vi "黑白棋.vi"() -> ()   [LabVIEW 2021]
panel:
  out "下棋者顏色":bool
  out "回合":dbl
  in  "停止":bool
  in  "開始":bool
  in  "Boolean 57":bool
  in  "Boolean 58":bool
  in  "Boolean 59":bool
  in  "Boolean 60":bool
  in  "Boolean 61":bool
  in  "Boolean 62":bool
  in  "Boolean 63":bool
  in  "Boolean 64":bool
  in  "Boolean 49":bool
  in  "Boolean 50":bool
  in  "Boolean 51":bool
  in  "Boolean 52":bool
  in  "Boolean 53":bool
  in  "Boolean 54":bool
  in  "Boolean 55":bool
  in  "Boolean 56":bool
  in  "Boolean 41":bool
  in  "Boolean 42":bool
  in  "Boolean 43":bool
  in  "Boolean 44":bool
  in  "Boolean 45":bool
  in  "Boolean 46":bool
  in  "Boolean 47":bool
  in  "Boolean 48":bool
  in  "Boolean 33":bool
  in  "Boolean 34":bool
  in  "Boolean 35":bool
  in  "Boolean 36":bool
  in  "Boolean 37":bool
  in  "Boolean 38":bool
  in  "Boolean 39":bool
  in  "Boolean 40":bool
  in  "Boolean 25":bool
  in  "Boolean 26":bool
  in  "Boolean 27":bool
  in  "Boolean 28":bool
  in  "Boolean 29":bool
  in  "Boolean 30":bool
  in  "Boolean 31":bool
  in  "Boolean 32":bool
  in  "Boolean 17":bool
  in  "Boolean 18":bool
  in  "Boolean 19":bool
  in  "Boolean 20":bool
  in  "Boolean 21":bool
  in  "Boolean 22":bool
  in  "Boolean 23":bool
  in  "Boolean 24":bool
  in  "Boolean 9":bool
  in  "Boolean 10":bool
  in  "Boolean 11":bool
  in  "Boolean 12":bool
  in  "Boolean 13":bool
  in  "Boolean 14":bool
  in  "Boolean 15":bool
  in  "Boolean 16":bool
  in  "Boolean 8":bool
  in  "Boolean 7":bool
  in  "Boolean 6":bool
  in  "Boolean 5":bool
  in  "Boolean 4":bool
  in  "Boolean 3":bool
  in  "Boolean 2":bool
  in  "Boolean":bool
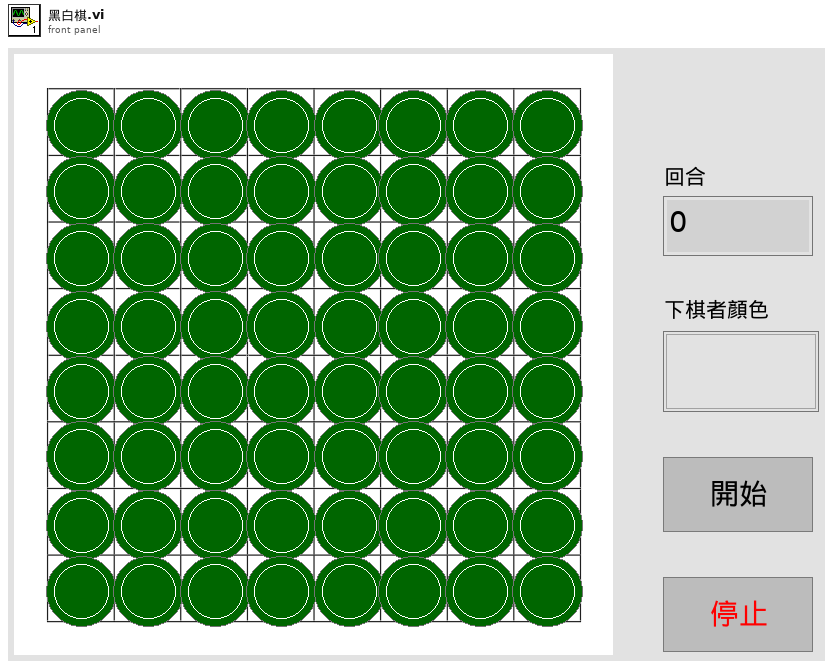
[diagram p1: front panel]
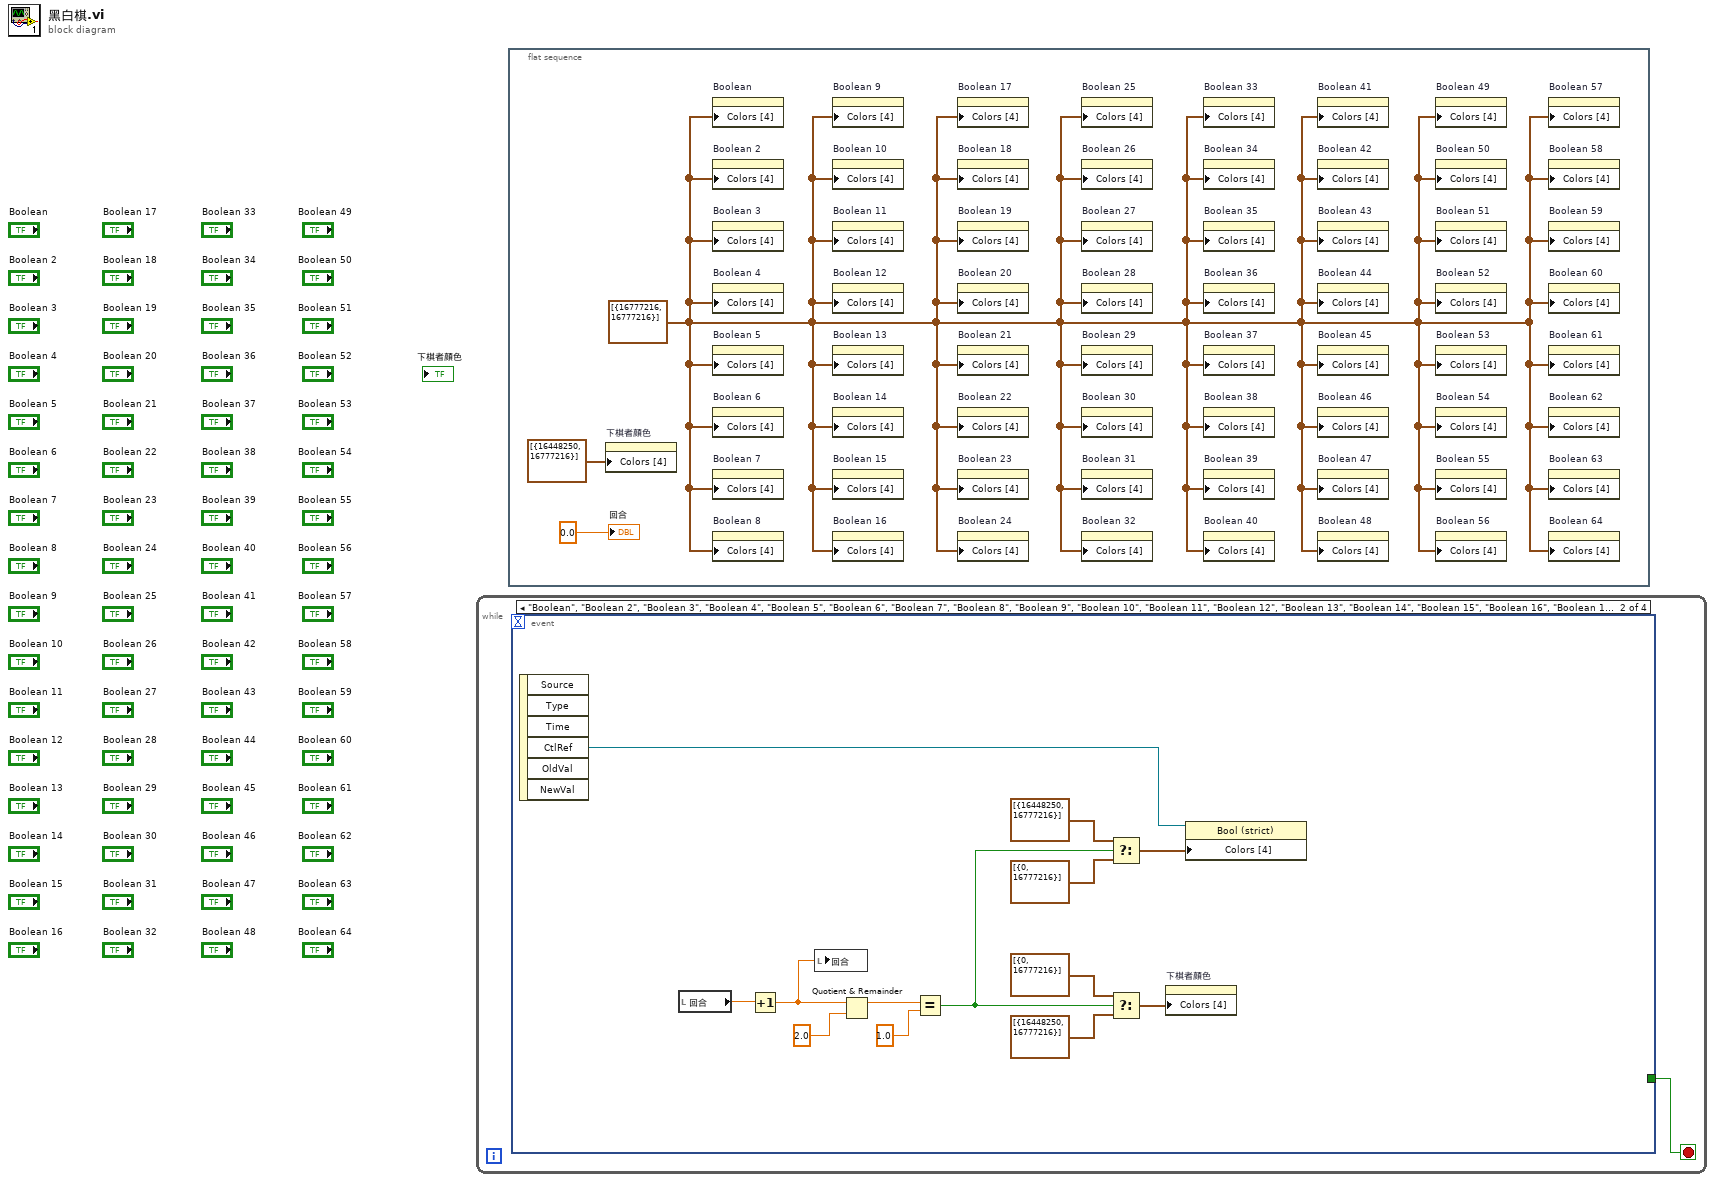
[diagram p0: block diagram]
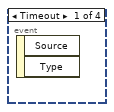
[diagram p2: hidden frame]
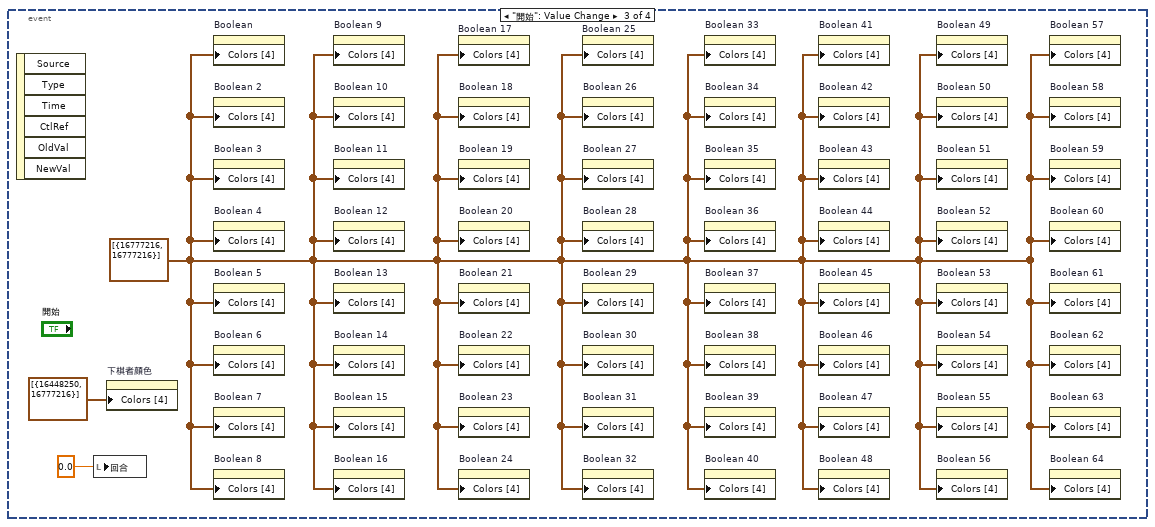
[diagram p3: hidden frame]
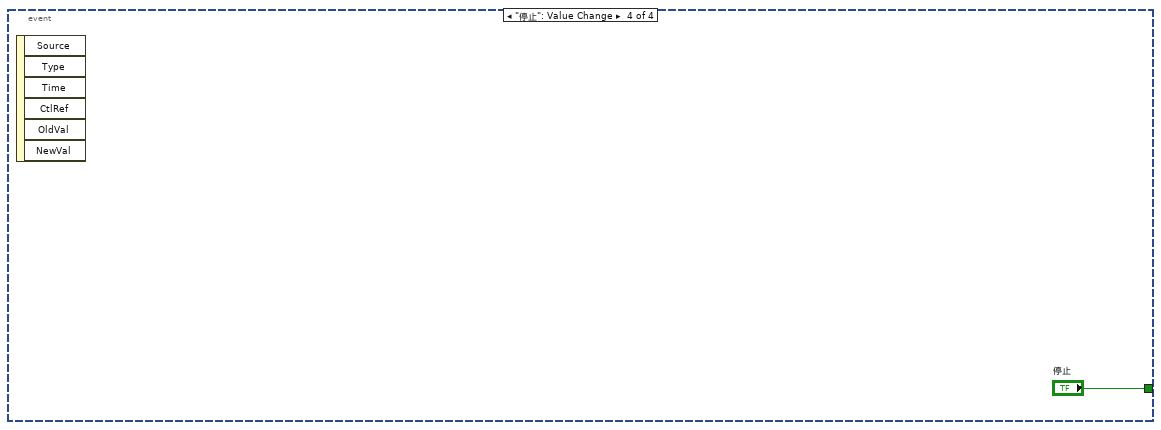
[diagram p4: hidden frame]
diagram:
  n1 = while {
    stop <- w1 stop-if-true
    n2 = event shown="[1] \"Boolean\", \"Boolean 2\", \"Boolean 3\", \"Boolean 4\", \"Boolean 5\", \"Boolean 6\", \"Boolean 7\", \"Boolean 8\", \"Boolean 9\", \"Boolean 10\", \"Boolean 11\", \"Boolean 12\", \"Boolean 13\", \"Boolean 14\", \"Boolean 15\", \"Boolean 16\", \"Boolean 17\", \"Boolean 18\", \"Boolean 19\", \"Boolean 20\", \"Boolean 21\", \"Boolean 22\", \"Boolean 23\", \"Boolean 24\", \"Boolean 25\", \"Boolean 26\", \"Boolean 27\", \"Boolean 28\", \"Boolean 29\", \"Boolean 30\", \"Boolean 31\", \"Boolean 32\", \"Boolean 33\", \"Boolean 34\", \"Boolean 35\", \"Boolean 36\", \"Boolean 37\", \"Boolean 38\", \"Boolean 39\", \"Boolean 40\", \"Boolean 41\", \"Boolean 42\", \"Boolean 43\", \"Boolean 44\", \"Boolean 45\", \"Boolean 46\", \"Boolean 47\", \"Boolean 48\", \"Boolean 49\", \"Boolean 50\", \"Boolean 51\", \"Boolean 52\", \"Boolean 53\", \"Boolean 54\", \"Boolean 55\", \"Boolean 56\", \"Boolean 57\", \"Boolean 58\", \"Boolean 59\", \"Boolean 60\", \"Boolean 61\", \"Boolean 62\", \"Boolean 63\", \"Boolean 64\": Value Change" {
      selector: _ -> [_ _ _ _]
      dyn-events: _ -> [_ _ _ _]
      timeout: _ -> [_ _ _ _]
      tunnel: [_ _ _ "停止"] -> w1
      event Timeout {
        n3 = event-data() -> ()  [unwired: 1 in, 2 out]
      }
      event "Boolean", "Boolean 2", "Boolean 3", "Boolean 4", "Boolean 5", "Boolean 6", "Boolean 7", "Boolean 8", "Boolean 9", "Boolean 10", "Boolean 11", "Boolean 12", "Boolean 13", "Boolean 14", "Boolean 15", "Boolean 16", "Boolean 17", "Boolean 18", "Boolean 19", "Boolean 20", "Boolean 21", "Boolean 22", "Boolean 23", "Boolean 24", "Boolean 25", "Boolean 26", "Boolean 27", "Boolean 28", "Boolean 29", "Boolean 30", "Boolean 31", "Boolean 32", "Boolean 33", "Boolean 34", "Boolean 35", "Boolean 36", "Boolean 37", "Boolean 38", "Boolean 39", "Boolean 40", "Boolean 41", "Boolean 42", "Boolean 43", "Boolean 44", "Boolean 45", "Boolean 46", "Boolean 47", "Boolean 48", "Boolean 49", "Boolean 50", "Boolean 51", "Boolean 52", "Boolean 53", "Boolean 54", "Boolean 55", "Boolean 56", "Boolean 57", "Boolean 58", "Boolean 59", "Boolean 60", "Boolean 61", "Boolean 62", "Boolean 63", "Boolean 64": Value Change {
        n4 = event-data() -> ("CtlRef"=w2:refnum<vi>)  [unwired: 1 in, 5 out]
        n5 = local read "回合"() -> (w14:dbl)
        n6 = Increment(x=w14) -> (x+1=w12:dbl)
        n7 = local write "回合"(w12) -> ()
        n8 = Quotient & Remainder(x=w12, y=2.0) -> (x-y*floor(x/y)=w11:dbl)  [unwired: 1 out]
        n9 = Equal?(x=w11, y=1.0) -> (x = y?=w3:bool)
        n10 = Select(t=cluster{u32, u32}[] [{16448250, 16777216}] ("Colors [4]"), s=w3, f=cluster{u32, u32}[] [{0, 16777216}] ("Colors [4]")) -> (s? t:f=w4:cluster{u32, u32}[])
        n11 = Select(t=cluster{u32, u32}[] [{0, 16777216}] ("Colors [4]"), s=w3, f=cluster{u32, u32}[] [{16448250, 16777216}] ("Colors [4]")) -> (s? t:f=w7:cluster{u32, u32}[])
        n12 = property on="下棋者顏色" class="Bool (strict)"("Colors [4]"=w7) -> ()  [unwired: 2 in, 2 out]
        n13 = property class="Bool (strict)"(reference=w2, "Colors [4]"=w4) -> ()  [unwired: 1 in, 2 out]
      }
      event "開始": Value Change {
        w15 = cluster{u32, u32}[] [{16777216, 16777216}] ("Colors [4]")
        n14 = event-data() -> ()  [unwired: 1 in, 6 out]
        n15 = local write "回合"(0.0 ("回合")) -> ()
        n16 = property on="下棋者顏色" class="Bool (strict)"("Colors [4]"=cluster{u32, u32}[] [{16448250, 16777216}]) -> ()  [unwired: 2 in, 2 out]
        n17 = property on="Boolean" class="Bool (strict)"("Colors [4]"=w15) -> ()  [unwired: 2 in, 2 out]
        n18 = property on="Boolean 2" class="Bool (strict)"("Colors [4]"=w15) -> ()  [unwired: 2 in, 2 out]
        n19 = property on="Boolean 3" class="Bool (strict)"("Colors [4]"=w15) -> ()  [unwired: 2 in, 2 out]
        n20 = property on="Boolean 4" class="Bool (strict)"("Colors [4]"=w15) -> ()  [unwired: 2 in, 2 out]
        n21 = property on="Boolean 5" class="Bool (strict)"("Colors [4]"=w15) -> ()  [unwired: 2 in, 2 out]
        n22 = property on="Boolean 6" class="Bool (strict)"("Colors [4]"=w15) -> ()  [unwired: 2 in, 2 out]
        n23 = property on="Boolean 7" class="Bool (strict)"("Colors [4]"=w15) -> ()  [unwired: 2 in, 2 out]
        n24 = property on="Boolean 8" class="Bool (strict)"("Colors [4]"=w15) -> ()  [unwired: 2 in, 2 out]
        n25 = property on="Boolean 9" class="Bool (strict)"("Colors [4]"=w15) -> ()  [unwired: 2 in, 2 out]
        n26 = property on="Boolean 10" class="Bool (strict)"("Colors [4]"=w15) -> ()  [unwired: 2 in, 2 out]
        n27 = property on="Boolean 11" class="Bool (strict)"("Colors [4]"=w15) -> ()  [unwired: 2 in, 2 out]
        n28 = property on="Boolean 12" class="Bool (strict)"("Colors [4]"=w15) -> ()  [unwired: 2 in, 2 out]
        n29 = property on="Boolean 13" class="Bool (strict)"("Colors [4]"=w15) -> ()  [unwired: 2 in, 2 out]
        n30 = property on="Boolean 14" class="Bool (strict)"("Colors [4]"=w15) -> ()  [unwired: 2 in, 2 out]
        n31 = property on="Boolean 15" class="Bool (strict)"("Colors [4]"=w15) -> ()  [unwired: 2 in, 2 out]
        n32 = property on="Boolean 16" class="Bool (strict)"("Colors [4]"=w15) -> ()  [unwired: 2 in, 2 out]
        n33 = property on="Boolean 17" class="Bool (strict)"("Colors [4]"=w15) -> ()  [unwired: 2 in, 2 out]
        n34 = property on="Boolean 18" class="Bool (strict)"("Colors [4]"=w15) -> ()  [unwired: 2 in, 2 out]
        n35 = property on="Boolean 19" class="Bool (strict)"("Colors [4]"=w15) -> ()  [unwired: 2 in, 2 out]
        n36 = property on="Boolean 20" class="Bool (strict)"("Colors [4]"=w15) -> ()  [unwired: 2 in, 2 out]
        n37 = property on="Boolean 21" class="Bool (strict)"("Colors [4]"=w15) -> ()  [unwired: 2 in, 2 out]
        n38 = property on="Boolean 22" class="Bool (strict)"("Colors [4]"=w15) -> ()  [unwired: 2 in, 2 out]
        n39 = property on="Boolean 23" class="Bool (strict)"("Colors [4]"=w15) -> ()  [unwired: 2 in, 2 out]
        n40 = property on="Boolean 24" class="Bool (strict)"("Colors [4]"=w15) -> ()  [unwired: 2 in, 2 out]
        n41 = property on="Boolean 25" class="Bool (strict)"("Colors [4]"=w15) -> ()  [unwired: 2 in, 2 out]
        n42 = property on="Boolean 26" class="Bool (strict)"("Colors [4]"=w15) -> ()  [unwired: 2 in, 2 out]
        n43 = property on="Boolean 27" class="Bool (strict)"("Colors [4]"=w15) -> ()  [unwired: 2 in, 2 out]
        n44 = property on="Boolean 28" class="Bool (strict)"("Colors [4]"=w15) -> ()  [unwired: 2 in, 2 out]
        n45 = property on="Boolean 29" class="Bool (strict)"("Colors [4]"=w15) -> ()  [unwired: 2 in, 2 out]
        n46 = property on="Boolean 30" class="Bool (strict)"("Colors [4]"=w15) -> ()  [unwired: 2 in, 2 out]
        n47 = property on="Boolean 31" class="Bool (strict)"("Colors [4]"=w15) -> ()  [unwired: 2 in, 2 out]
        n48 = property on="Boolean 32" class="Bool (strict)"("Colors [4]"=w15) -> ()  [unwired: 2 in, 2 out]
        n49 = property on="Boolean 33" class="Bool (strict)"("Colors [4]"=w15) -> ()  [unwired: 2 in, 2 out]
        n50 = property on="Boolean 34" class="Bool (strict)"("Colors [4]"=w15) -> ()  [unwired: 2 in, 2 out]
        n51 = property on="Boolean 35" class="Bool (strict)"("Colors [4]"=w15) -> ()  [unwired: 2 in, 2 out]
        n52 = property on="Boolean 36" class="Bool (strict)"("Colors [4]"=w15) -> ()  [unwired: 2 in, 2 out]
        n53 = property on="Boolean 37" class="Bool (strict)"("Colors [4]"=w15) -> ()  [unwired: 2 in, 2 out]
        n54 = property on="Boolean 38" class="Bool (strict)"("Colors [4]"=w15) -> ()  [unwired: 2 in, 2 out]
        n55 = property on="Boolean 39" class="Bool (strict)"("Colors [4]"=w15) -> ()  [unwired: 2 in, 2 out]
        n56 = property on="Boolean 40" class="Bool (strict)"("Colors [4]"=w15) -> ()  [unwired: 2 in, 2 out]
        n57 = property on="Boolean 41" class="Bool (strict)"("Colors [4]"=w15) -> ()  [unwired: 2 in, 2 out]
        n58 = property on="Boolean 42" class="Bool (strict)"("Colors [4]"=w15) -> ()  [unwired: 2 in, 2 out]
        n59 = property on="Boolean 43" class="Bool (strict)"("Colors [4]"=w15) -> ()  [unwired: 2 in, 2 out]
        n60 = property on="Boolean 44" class="Bool (strict)"("Colors [4]"=w15) -> ()  [unwired: 2 in, 2 out]
        n61 = property on="Boolean 45" class="Bool (strict)"("Colors [4]"=w15) -> ()  [unwired: 2 in, 2 out]
        n62 = property on="Boolean 46" class="Bool (strict)"("Colors [4]"=w15) -> ()  [unwired: 2 in, 2 out]
        n63 = property on="Boolean 47" class="Bool (strict)"("Colors [4]"=w15) -> ()  [unwired: 2 in, 2 out]
        n64 = property on="Boolean 48" class="Bool (strict)"("Colors [4]"=w15) -> ()  [unwired: 2 in, 2 out]
        n65 = property on="Boolean 49" class="Bool (strict)"("Colors [4]"=w15) -> ()  [unwired: 2 in, 2 out]
        n66 = property on="Boolean 50" class="Bool (strict)"("Colors [4]"=w15) -> ()  [unwired: 2 in, 2 out]
        n67 = property on="Boolean 51" class="Bool (strict)"("Colors [4]"=w15) -> ()  [unwired: 2 in, 2 out]
        n68 = property on="Boolean 52" class="Bool (strict)"("Colors [4]"=w15) -> ()  [unwired: 2 in, 2 out]
        n69 = property on="Boolean 53" class="Bool (strict)"("Colors [4]"=w15) -> ()  [unwired: 2 in, 2 out]
        n70 = property on="Boolean 54" class="Bool (strict)"("Colors [4]"=w15) -> ()  [unwired: 2 in, 2 out]
        n71 = property on="Boolean 55" class="Bool (strict)"("Colors [4]"=w15) -> ()  [unwired: 2 in, 2 out]
        n72 = property on="Boolean 56" class="Bool (strict)"("Colors [4]"=w15) -> ()  [unwired: 2 in, 2 out]
        n73 = property on="Boolean 57" class="Bool (strict)"("Colors [4]"=w15) -> ()  [unwired: 2 in, 2 out]
        n74 = property on="Boolean 58" class="Bool (strict)"("Colors [4]"=w15) -> ()  [unwired: 2 in, 2 out]
        n75 = property on="Boolean 59" class="Bool (strict)"("Colors [4]"=w15) -> ()  [unwired: 2 in, 2 out]
        n76 = property on="Boolean 60" class="Bool (strict)"("Colors [4]"=w15) -> ()  [unwired: 2 in, 2 out]
        n77 = property on="Boolean 61" class="Bool (strict)"("Colors [4]"=w15) -> ()  [unwired: 2 in, 2 out]
        n78 = property on="Boolean 62" class="Bool (strict)"("Colors [4]"=w15) -> ()  [unwired: 2 in, 2 out]
        n79 = property on="Boolean 63" class="Bool (strict)"("Colors [4]"=w15) -> ()  [unwired: 2 in, 2 out]
        n80 = property on="Boolean 64" class="Bool (strict)"("Colors [4]"=w15) -> ()  [unwired: 2 in, 2 out]
      }
      event "停止": Value Change {
        n81 = event-data() -> ()  [unwired: 1 in, 6 out]
      }
    }
  }
  n82 = flat-sequence {
    frame #0 {
      w21 = cluster{u32, u32}[] [{16777216, 16777216}] ("Colors [4]")
      n83 = property on="下棋者顏色" class="Bool (strict)"("Colors [4]"=cluster{u32, u32}[] [{16448250, 16777216}]) -> ()  [unwired: 2 in, 2 out]
      n84 = property on="Boolean" class="Bool (strict)"("Colors [4]"=w21) -> ()  [unwired: 2 in, 2 out]
      n85 = property on="Boolean 2" class="Bool (strict)"("Colors [4]"=w21) -> ()  [unwired: 2 in, 2 out]
      n86 = property on="Boolean 3" class="Bool (strict)"("Colors [4]"=w21) -> ()  [unwired: 2 in, 2 out]
      n87 = property on="Boolean 4" class="Bool (strict)"("Colors [4]"=w21) -> ()  [unwired: 2 in, 2 out]
      n88 = property on="Boolean 5" class="Bool (strict)"("Colors [4]"=w21) -> ()  [unwired: 2 in, 2 out]
      n89 = property on="Boolean 6" class="Bool (strict)"("Colors [4]"=w21) -> ()  [unwired: 2 in, 2 out]
      n90 = property on="Boolean 7" class="Bool (strict)"("Colors [4]"=w21) -> ()  [unwired: 2 in, 2 out]
      n91 = property on="Boolean 8" class="Bool (strict)"("Colors [4]"=w21) -> ()  [unwired: 2 in, 2 out]
      n92 = property on="Boolean 9" class="Bool (strict)"("Colors [4]"=w21) -> ()  [unwired: 2 in, 2 out]
      n93 = property on="Boolean 10" class="Bool (strict)"("Colors [4]"=w21) -> ()  [unwired: 2 in, 2 out]
      n94 = property on="Boolean 11" class="Bool (strict)"("Colors [4]"=w21) -> ()  [unwired: 2 in, 2 out]
      n95 = property on="Boolean 12" class="Bool (strict)"("Colors [4]"=w21) -> ()  [unwired: 2 in, 2 out]
      n96 = property on="Boolean 13" class="Bool (strict)"("Colors [4]"=w21) -> ()  [unwired: 2 in, 2 out]
      n97 = property on="Boolean 14" class="Bool (strict)"("Colors [4]"=w21) -> ()  [unwired: 2 in, 2 out]
      n98 = property on="Boolean 15" class="Bool (strict)"("Colors [4]"=w21) -> ()  [unwired: 2 in, 2 out]
      n99 = property on="Boolean 16" class="Bool (strict)"("Colors [4]"=w21) -> ()  [unwired: 2 in, 2 out]
      n100 = property on="Boolean 17" class="Bool (strict)"("Colors [4]"=w21) -> ()  [unwired: 2 in, 2 out]
      n101 = property on="Boolean 18" class="Bool (strict)"("Colors [4]"=w21) -> ()  [unwired: 2 in, 2 out]
      n102 = property on="Boolean 19" class="Bool (strict)"("Colors [4]"=w21) -> ()  [unwired: 2 in, 2 out]
      n103 = property on="Boolean 20" class="Bool (strict)"("Colors [4]"=w21) -> ()  [unwired: 2 in, 2 out]
      n104 = property on="Boolean 21" class="Bool (strict)"("Colors [4]"=w21) -> ()  [unwired: 2 in, 2 out]
      n105 = property on="Boolean 22" class="Bool (strict)"("Colors [4]"=w21) -> ()  [unwired: 2 in, 2 out]
      n106 = property on="Boolean 23" class="Bool (strict)"("Colors [4]"=w21) -> ()  [unwired: 2 in, 2 out]
      n107 = property on="Boolean 24" class="Bool (strict)"("Colors [4]"=w21) -> ()  [unwired: 2 in, 2 out]
      n108 = property on="Boolean 25" class="Bool (strict)"("Colors [4]"=w21) -> ()  [unwired: 2 in, 2 out]
      n109 = property on="Boolean 26" class="Bool (strict)"("Colors [4]"=w21) -> ()  [unwired: 2 in, 2 out]
      n110 = property on="Boolean 27" class="Bool (strict)"("Colors [4]"=w21) -> ()  [unwired: 2 in, 2 out]
      n111 = property on="Boolean 28" class="Bool (strict)"("Colors [4]"=w21) -> ()  [unwired: 2 in, 2 out]
      n112 = property on="Boolean 29" class="Bool (strict)"("Colors [4]"=w21) -> ()  [unwired: 2 in, 2 out]
      n113 = property on="Boolean 30" class="Bool (strict)"("Colors [4]"=w21) -> ()  [unwired: 2 in, 2 out]
      n114 = property on="Boolean 31" class="Bool (strict)"("Colors [4]"=w21) -> ()  [unwired: 2 in, 2 out]
      n115 = property on="Boolean 32" class="Bool (strict)"("Colors [4]"=w21) -> ()  [unwired: 2 in, 2 out]
      n116 = property on="Boolean 33" class="Bool (strict)"("Colors [4]"=w21) -> ()  [unwired: 2 in, 2 out]
      n117 = property on="Boolean 34" class="Bool (strict)"("Colors [4]"=w21) -> ()  [unwired: 2 in, 2 out]
      n118 = property on="Boolean 35" class="Bool (strict)"("Colors [4]"=w21) -> ()  [unwired: 2 in, 2 out]
      n119 = property on="Boolean 36" class="Bool (strict)"("Colors [4]"=w21) -> ()  [unwired: 2 in, 2 out]
      n120 = property on="Boolean 37" class="Bool (strict)"("Colors [4]"=w21) -> ()  [unwired: 2 in, 2 out]
      n121 = property on="Boolean 38" class="Bool (strict)"("Colors [4]"=w21) -> ()  [unwired: 2 in, 2 out]
      n122 = property on="Boolean 39" class="Bool (strict)"("Colors [4]"=w21) -> ()  [unwired: 2 in, 2 out]
      n123 = property on="Boolean 40" class="Bool (strict)"("Colors [4]"=w21) -> ()  [unwired: 2 in, 2 out]
      n124 = property on="Boolean 41" class="Bool (strict)"("Colors [4]"=w21) -> ()  [unwired: 2 in, 2 out]
      n125 = property on="Boolean 42" class="Bool (strict)"("Colors [4]"=w21) -> ()  [unwired: 2 in, 2 out]
      n126 = property on="Boolean 43" class="Bool (strict)"("Colors [4]"=w21) -> ()  [unwired: 2 in, 2 out]
      n127 = property on="Boolean 44" class="Bool (strict)"("Colors [4]"=w21) -> ()  [unwired: 2 in, 2 out]
      n128 = property on="Boolean 45" class="Bool (strict)"("Colors [4]"=w21) -> ()  [unwired: 2 in, 2 out]
      n129 = property on="Boolean 46" class="Bool (strict)"("Colors [4]"=w21) -> ()  [unwired: 2 in, 2 out]
      n130 = property on="Boolean 47" class="Bool (strict)"("Colors [4]"=w21) -> ()  [unwired: 2 in, 2 out]
      n131 = property on="Boolean 48" class="Bool (strict)"("Colors [4]"=w21) -> ()  [unwired: 2 in, 2 out]
      n132 = property on="Boolean 49" class="Bool (strict)"("Colors [4]"=w21) -> ()  [unwired: 2 in, 2 out]
      n133 = property on="Boolean 50" class="Bool (strict)"("Colors [4]"=w21) -> ()  [unwired: 2 in, 2 out]
      n134 = property on="Boolean 51" class="Bool (strict)"("Colors [4]"=w21) -> ()  [unwired: 2 in, 2 out]
      n135 = property on="Boolean 52" class="Bool (strict)"("Colors [4]"=w21) -> ()  [unwired: 2 in, 2 out]
      n136 = property on="Boolean 53" class="Bool (strict)"("Colors [4]"=w21) -> ()  [unwired: 2 in, 2 out]
      n137 = property on="Boolean 54" class="Bool (strict)"("Colors [4]"=w21) -> ()  [unwired: 2 in, 2 out]
      n138 = property on="Boolean 55" class="Bool (strict)"("Colors [4]"=w21) -> ()  [unwired: 2 in, 2 out]
      n139 = property on="Boolean 56" class="Bool (strict)"("Colors [4]"=w21) -> ()  [unwired: 2 in, 2 out]
      n140 = property on="Boolean 57" class="Bool (strict)"("Colors [4]"=w21) -> ()  [unwired: 2 in, 2 out]
      n141 = property on="Boolean 58" class="Bool (strict)"("Colors [4]"=w21) -> ()  [unwired: 2 in, 2 out]
      n142 = property on="Boolean 59" class="Bool (strict)"("Colors [4]"=w21) -> ()  [unwired: 2 in, 2 out]
      n143 = property on="Boolean 60" class="Bool (strict)"("Colors [4]"=w21) -> ()  [unwired: 2 in, 2 out]
      n144 = property on="Boolean 61" class="Bool (strict)"("Colors [4]"=w21) -> ()  [unwired: 2 in, 2 out]
      n145 = property on="Boolean 62" class="Bool (strict)"("Colors [4]"=w21) -> ()  [unwired: 2 in, 2 out]
      n146 = property on="Boolean 63" class="Bool (strict)"("Colors [4]"=w21) -> ()  [unwired: 2 in, 2 out]
      n147 = property on="Boolean 64" class="Bool (strict)"("Colors [4]"=w21) -> ()  [unwired: 2 in, 2 out]
      "回合" <- 0.0 ("回合")
    }
  }
